vi "Set ni_bus_monitor_api_StreamBusReply.vi"(7 "Complete Call (T)":bool=TRUE, 8 "error in (no error)":errorcluster, 10 "package_templatemessage":T1, 11 "gRPCid":T7) -> (0 "error out":errorcluster)   [LabVIEW 2025, in "bus_monitor_server.lvlib"]
uses:
  bus_monitor_server.lvlib
  <vilib>/gRPC/LabVIEW gRPC Library/Shared/grpcId.ctl
  ni_bus_monitor_api_StreamBusReply.ctl
  ni_bus_monitor_api_CanCommState.ctl
  ni_bus_monitor_api_CommState.ctl
  ni_bus_monitor_api_LastCommError.ctl
  ni_bus_monitor_api_Frame.ctl
  ni_bus_monitor_api_ErrorInfo.ctl
  ni_bus_monitor_api_StreamBusReply_Flat.ctl
  ni_bus_monitor_api_CanCommState_Flat.ctl
  ni_bus_monitor_api_Frame_Flat.ctl
  ni_bus_monitor_api_ErrorInfo_Flat.ctl
  dcc74a39-081a-4bdd-860b-8ed792803c96.vi
  RichToFlatni_bus_monitor_api_CanCommState.vi
  RichToFlatni_bus_monitor_api_Frame.vi
  RichToFlatni_bus_monitor_api_ErrorInfo.vi
  <vilib>/gRPC/LabVIEW gRPC Library/Shared/TranslateGrpcError.vi
  <vilib>/gRPC/LabVIEW gRPC Library/Server API/Server/Get Server DLL Path.vi
  <vilib>/Utility/error.llb/Error Cluster From Error Code.vi
  <vilib>/gRPC/LabVIEW gRPC Library/grpc-lvsupport-release.lvlib
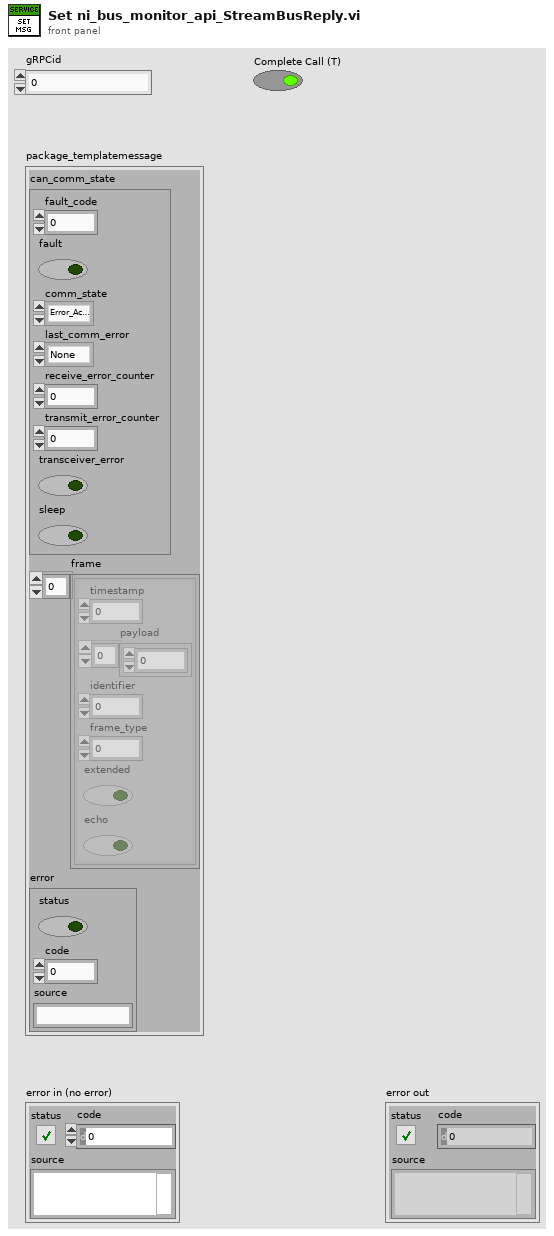
[diagram p1: front panel]
types:
  T1 = typedef "bus_monitor_server.lvlib/ni_bus_monitor_api_StreamBusReply.ctl" = cluster{"can_comm_state":T2, "frame":T5[], "error":T6}
  T2 = typedef "bus_monitor_server.lvlib/ni_bus_monitor_api_CanCommState.ctl" = cluster{"fault_code":i32, "fault":bool, "comm_state":T3, "last_comm_error":T4, "receive_error_counter":u32, "transmit_error_counter":u32, "transceiver_error":bool, "sleep":bool}
  T3 = typedef "bus_monitor_server.lvlib/ni_bus_monitor_api_CommState.ctl" = enum32{"Error_Active", "Error_Passive", "Bus_Off", "Init"}
  T4 = typedef "bus_monitor_server.lvlib/ni_bus_monitor_api_LastCommError.ctl" = enum32{"None", "Stuff", "Form", "ACK", "Bit1", "Bit0", "CRC"}
  T5 = typedef "bus_monitor_server.lvlib/ni_bus_monitor_api_Frame.ctl" = cluster{"timestamp":dbl, "payload":u8[], "identifier":u32, "frame_type":u32, "extended":bool, "echo":bool}
  T6 = typedef "bus_monitor_server.lvlib/ni_bus_monitor_api_ErrorInfo.ctl" = errorcluster
  T7 = typedef "grpc-lvsupport-release.lvlib/grpcId.ctl" = u64
  T8 = typedef "bus_monitor_server.lvlib/ni_bus_monitor_api_StreamBusReply_Flat.ctl" = cluster{"can_comm_state":T9, "frame":T10[], "error":T11}
  T9 = typedef "bus_monitor_server.lvlib/ni_bus_monitor_api_CanCommState_Flat.ctl" = cluster{"fault_code":i32, "fault":bool, "comm_state":T3, "last_comm_error":T4, "receive_error_counter":u32, "transmit_error_counter":u32, "transceiver_error":bool, "sleep":bool}
  T10 = typedef "bus_monitor_server.lvlib/ni_bus_monitor_api_Frame_Flat.ctl" = cluster{"timestamp":dbl, "payload":u8[], "identifier":u32, "frame_type":u32, "extended":bool, "echo":bool}
  T11 = typedef "bus_monitor_server.lvlib/ni_bus_monitor_api_ErrorInfo_Flat.ctl" = errorcluster
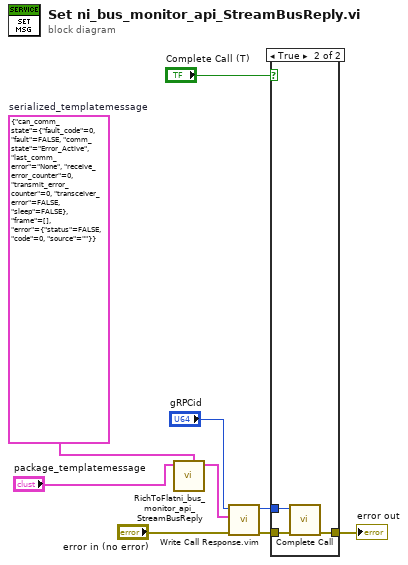
[diagram p0: block diagram]
diagram:
  w2 = T8 {"can_comm_state"={"fault_code"=0, "fault"=FALSE, "comm_state"=enum."Error_Active", "last_comm_error"=enum."None", "receive_error_counter"=0, "transmit_error_counter"=0, "transceiver_error"=FALSE, "sleep"=FALSE}, "frame"=[], "error"={"status"=FALSE, "code"=0, "source"=""}}  # serialized_templatemessage
  n1 = call "RichToFlatni_bus_monitor_api_StreamBusReply.vi"("OutputClusterType"=w2, "InputCluster"="package_templatemessage") -> ("OutputCluster"=w1:T8)  [unwired: 9 in]
  n2 = call "Write Call Response.vim"("error in"="error in (no error)", "Response Data"=w1, "gRPCid in"="gRPCid") -> ("error out"=w6:errorcluster, "gRPCid out"=w7:T7)  [unwired: 7 in]
  n3 = case shown="True" "Complete Call (T)" {
    tunnel: [w10 w13] -> w9
    tunnel: w7 -> [_ w12]
    tunnel: w6 -> [w10 w11]
    frame False {
    }
    frame True {
      n4 = call <vilib>:"Complete Call.vi"("gRPCid"=w12, "error in"=w11) -> ("error out"=w13:errorcluster)  [unwired: 8 in]
    }
  }
  "error out" <- w9
